vi "Read Meta Data (UDP Ref).vi"(6 "options":T4={"ignore timeout error"=TRUE, "timeout ms (1000)"=1000, "max size (548)"=548}, 8 "error in":errorcluster, 11 "connection ID":refnum<k16>) -> (0 "error out":errorcluster, 1 "meta data":T1[](array[typedef]), 3 "connection info out":T2, 4 "data info":T3)   [LabVIEW 2010, in "NI STM.lvlib"]
doc: "This VI reads the meta data information from a remote computer. Use this VI to retrieve the variable names and types that a remote computer exports.\n\nThis VI parses the data and returns a cluster containing the meta data information."
uses:
  NI STM.lvlib
  UDP Read Options.ctl
  UDP Data Info.ctl
  UDP Connection Info.ctl
  SubVIs/MetaDataElement.ctl
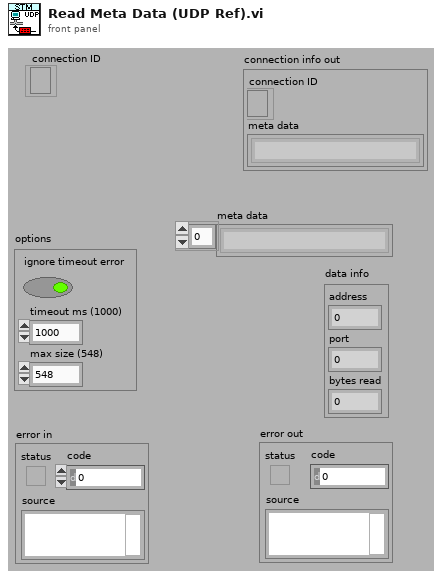
[diagram p1: front panel]
types:
  T1 = typedef "NI STM.lvlib/MetaDataElement.ctl" = string
  T2 = typedef "NI STM.lvlib/UDP Connection Info.ctl" = cluster{"connection ID":refnum<k16>, "meta data":T1[]}
  T3 = typedef "NI STM.lvlib/UDP Data Info.ctl" = cluster{"address":u32, "port":u16, "bytes read":i32}
  T4 = typedef "NI STM.lvlib/UDP Read Options.ctl" = cluster{"ignore timeout error":bool, "timeout ms (1000)":i32, "max size (548)":i32}
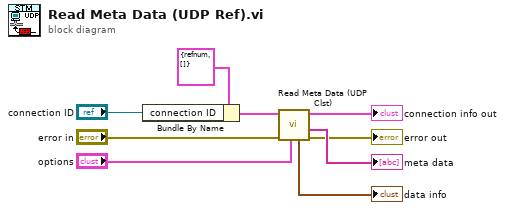
[diagram p0: block diagram]
diagram:
  n1 = Bundle By Name(cluster=T2 {"connection ID"=refnum, "meta data"=[]} ("Connection Info Out"), "connection ID"="connection ID") -> (w7:T2)
  n2 = call "Read Meta Data (UDP Clst).vi"("options"="options", "error in"="error in", "connection info in"=w7) -> ("error out"=→"error out":errorcluster, "meta data"=→"meta data":T1[], "connection info out"=→"connection info out":T2, "data info"=→"data info":T3)  [unwired: 5 in]
